vi "ErrorCheckHWI.vi"(8 "error in (no error)":errorcluster, 11 "DDS in":refnum<class "DDS.lvclass">) -> (0 "error out":errorcluster, 3 "DDS out":refnum<class "DDS.lvclass">)   [LabVIEW 2013, in "DDS.lvclass"]
uses:
  DDS.lvclass
  DDS.lvclass/DDS.ctl
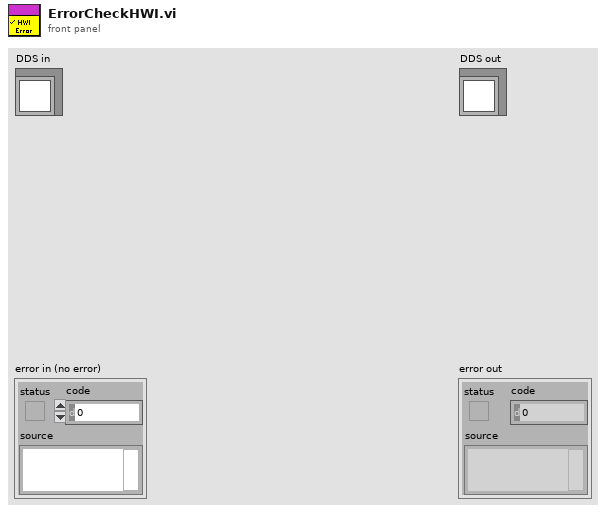
[diagram p1: front panel]
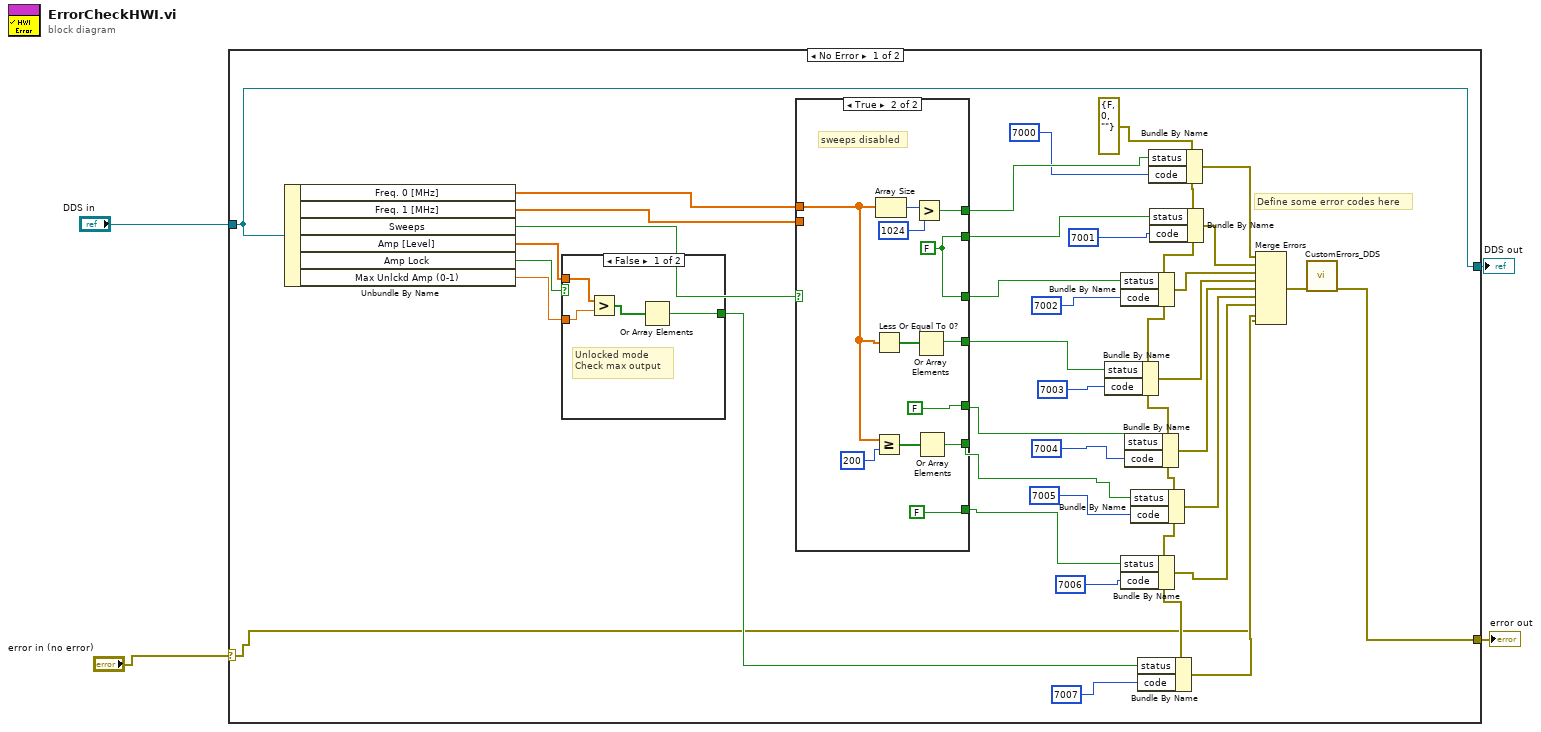
[diagram p0: block diagram]
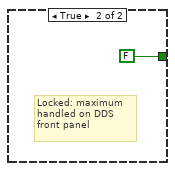
[diagram p2: hidden frame]
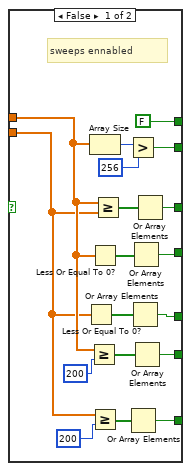
[diagram p3: hidden frame]
diagram:
  n1 = case shown="No Error" "error in (no error)" {
    selector: "error in (no error)" -> [w5 w75]
    tunnel: "DDS in" -> [w36 w76]
    tunnel: [w36 w76] -> w2
    tunnel: [w31 w75] -> w1
    frame No Error {
      w6 = errorcluster {"status"=FALSE, "code"=0, "source"=""} ("error constant")
      # "Define some error codes here"
      n2 = Unbundle By Name(w36) -> ("Freq. 0 [MHz]"=w38:dbl[], "Freq. 1 [MHz]"=w37:dbl[], "Sweeps"=w39:bool, "Amp [Level]"=w33:dbl[], "Amp Lock"=w35:bool, "Max Unlckd Amp (0-1)"=w34:dbl)
      n3 = case shown="False" w35 {
        tunnel: w34 -> [w43 _]
        tunnel: w33 -> [w42 _]
        tunnel: [w40 FALSE] -> w26
        frame False {
          # "Unlocked mode\nCheck max output"
          n4 = Greater?(x=w42, y=w43) -> (0:w41:bool[])
          n5 = Or Array Elements(Boolean array=w41) -> (logical OR=w40:bool)
        }
        frame True {
          # "Locked: maximum\nhandled on DDS\nfront panel"
        }
      }
      n6 = case shown="True" w39 {
        tunnel: [w45 w66] -> w19
        tunnel: w38 -> [w54 w65]
        tunnel: w37 -> [w51 _]
        tunnel: [FALSE w72] -> w30
        tunnel: [w59 w66] -> w22
        tunnel: [w57 w63] -> w17
        tunnel: [w55 FALSE] -> w15
        tunnel: [w49 w68] -> w12
        tunnel: [w47 FALSE] -> w8
        frame False {
          # "sweeps ennabled"
          n7 = Less Or Equal To 0?(x=w51) -> (x <= 0?=w56:bool[])
          n8 = Greater Or Equal?(x=w54, y=200) -> (x >= y?=w50:bool[])
          n9 = Array Size(array=w54) -> (size(s)=w61:i32)
          n10 = Less Or Equal To 0?(x=w54) -> (x <= 0?=w58:bool[])
          n11 = Greater Or Equal?(x=w51, y=200) -> (x >= y?=w48:bool[])
          n12 = Greater Or Equal?(x=w54, y=w51) -> (x >= y?=w46:bool[])
          n13 = Greater?(x=w61, y=256) -> (0:w59:bool)
          n14 = Or Array Elements(Boolean array=w48) -> (logical OR=w47:bool)
          n15 = Or Array Elements(Boolean array=w56) -> (logical OR=w55:bool)
          n16 = Or Array Elements(Boolean array=w58) -> (logical OR=w57:bool)
          n17 = Or Array Elements(Boolean array=w50) -> (logical OR=w49:bool)
          n18 = Or Array Elements(Boolean array=w46) -> (logical OR=w45:bool)
        }
        frame True {
          w66 = FALSE
          # "sweeps disabled"
          n19 = Less Or Equal To 0?(x=w65) -> (x <= 0?=w64:bool[])
          n20 = Greater Or Equal?(x=w65, y=200) -> (x >= y?=w70:bool[])
          n21 = Array Size(array=w65) -> (size(s)=w74:i32)
          n22 = Greater?(x=w74, y=1024) -> (0:w72:bool)
          n23 = Or Array Elements(Boolean array=w64) -> (logical OR=w63:bool)
          n24 = Or Array Elements(Boolean array=w70) -> (logical OR=w68:bool)
        }
      }
      n25 = Bundle By Name(cluster=w6, "status"=w17, "code"=7003 ("error code (0)")) -> (w18:errorcluster)
      n26 = Bundle By Name(cluster=w6, "status"=w19, "code"=7002 ("error code (0)")) -> (w21:errorcluster)
      n27 = Bundle By Name(cluster=w6, "status"=w8, "code"=7006 ("error code (0)")) -> (w9:errorcluster)
      n28 = Bundle By Name(cluster=w6, "status"=w15, "code"=7004 ("error code (0)")) -> (w13:errorcluster)
      n29 = Bundle By Name(cluster=w6, "status"=w12, "code"=7005 ("error code (0)")) -> (w10:errorcluster)
      n30 = Bundle By Name(cluster=w6, "status"=w26, "code"=7007 ("error code (0)")) -> (w25:errorcluster)
      n31 = Bundle By Name(cluster=w6, "status"=w30, "code"=7000 ("error code (0)")) -> (w28:errorcluster)
      n32 = Bundle By Name(cluster=w6, "status"=w22, "code"=7001 ("error code (0)")) -> (w24:errorcluster)
      n33 = Merge Errors(w28, w24, w21, w18, w13, w10, w9, w25, w5) -> (w32:errorcluster)
      n34 = call "CustomErrors_DDS.vi"("error in (no error)"=w32) -> ("error out"=w31:errorcluster)  [unwired: 10 in]
    }
    frame Error {
    }
  }
  "error out" <- w1
  "DDS out" <- w2
